vi "PDLM_GetBurst.vi"(8 "error in (no error)":errorcluster, 11 "USBIdx":i32) -> (0 "error out":errorcluster, 1 "PeriodLen":u32, 2 "BurstLen":u32, 3 "return type":i32)   [LabVIEW 2017]
uses:
  PDLM_DllPath_global.vi
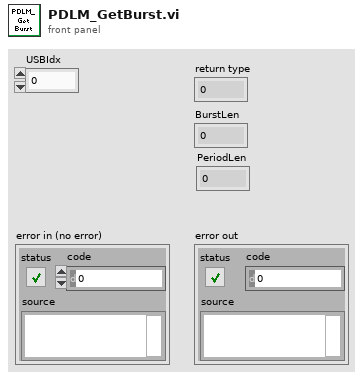
[diagram p1: front panel]
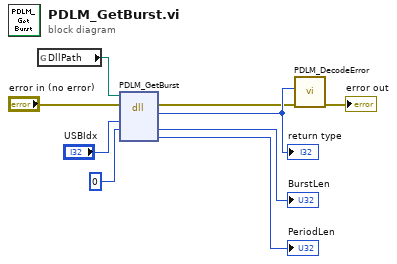
[diagram p0: block diagram]
diagram:
  n1 = global read "PDLM_DllPath_global.vi" "DllPath"() -> (w5:path)
  n2 = dll-call lib="M:/_dev/progs/LabVIEW/_lib/PQ/Taiko/pdlm_lib.dll" fn="PDLM_GetBurst"(path in=w5, error in="error in (no error)", "USBIdx"="USBIdx", "BurstLen"=u32 0 ("mode")) -> (error out=w7:errorcluster, "return type"=w8:i32, "BurstLen"=→"BurstLen":u32, "PeriodLen"=→"PeriodLen":u32)  [unwired: 3 in, 1 out]
  "return type" <- w8
  n3 = call "PDLM_DecodeError.vi"("error in (no error)"=w7, "code"=w8) -> ("error out"=→"error out":errorcluster)  [unwired: 7 in, 2 out]
